vi "Init MFCs Server.vi"(8 "error in":errorcluster) -> (0 "error out":errorcluster, 3 "Alicats":refnum<class "Alicat Device.lvclass">[](array[class]))   [LabVIEW 2015]
uses:
  Devices/Alicat/Session Based/Alicat Device.lvclass
  Controls/MFC Address.ctl
  Reusable/Session APIs/File Access/Config Data/Config Data.lvclass
  Reusable/Session APIs/Serial/Serial Session.lvclass
  Reusable/Session APIs/File Access/Config Data/Config Session.ctl
  Reusable/Session Log/System Log.lvclass
  Reusable/Session Log/System Log.lvclass/System Log.ctl
  Reusable/Session APIs/File Access/Config Data/Config Data.lvclass/Config Data.ctl
  Reusable/Session APIs/Text Communication/Text Device Session.lvclass/Text Device Session.ctl
  Devices/Configurable Device/Configurable Device.lvclass/Configurable Device.ctl
  Devices/Alicat/Session Based/Alicat Device.lvclass/Alicat Device.ctl
  Reusable/Session APIs/Text Communication/Write hSysLog.vi
  Devices/Configurable Device/Write Handle.vi
  Devices/Alicat/Session Based/Accessors/Write Session Handle.vi
  Devices/Alicat/Session Based/Accessors/Write ID.vi
  Reusable/Session Log/Accessors/Write Main Path.vi
  <vilib>/Utility/config.llb/Read Key (String).vi
  <userlib>/_Session Fwk/Session - Root.lvclass
  <vilib>/Utility/config.llb/NI_LVConfig.lvlib
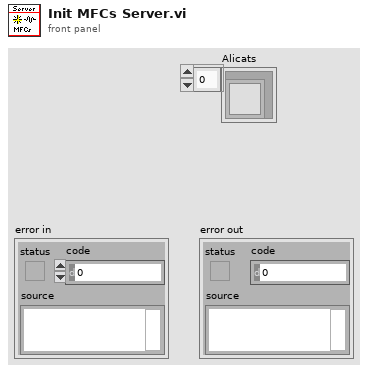
[diagram p1: front panel]
types:
  T1 = typedef "Config Data.lvclass/Config Session.ctl" = refnum<data-value>
  T2 = typedef "MFC Address.ctl" = enum16{"CRDS Purge", "CRDS Thermodenuded", "CRDS Dry", "CRDS Med RH", "CRDS High RH", "PAS Ch 1", "PAS Ch 2", "PAS Ch3", "PAS Ch 4", "PAS Ch 5", "CLAP", "O3", "Pinlet"}
  T3 = typedef "Session - Root.lvclass/Session Handle.ctl" = refnum<data-value>
  T4 = typedef "NI_LVConfig.lvlib/Config Data RefNum.ctl" = refnum<k1>
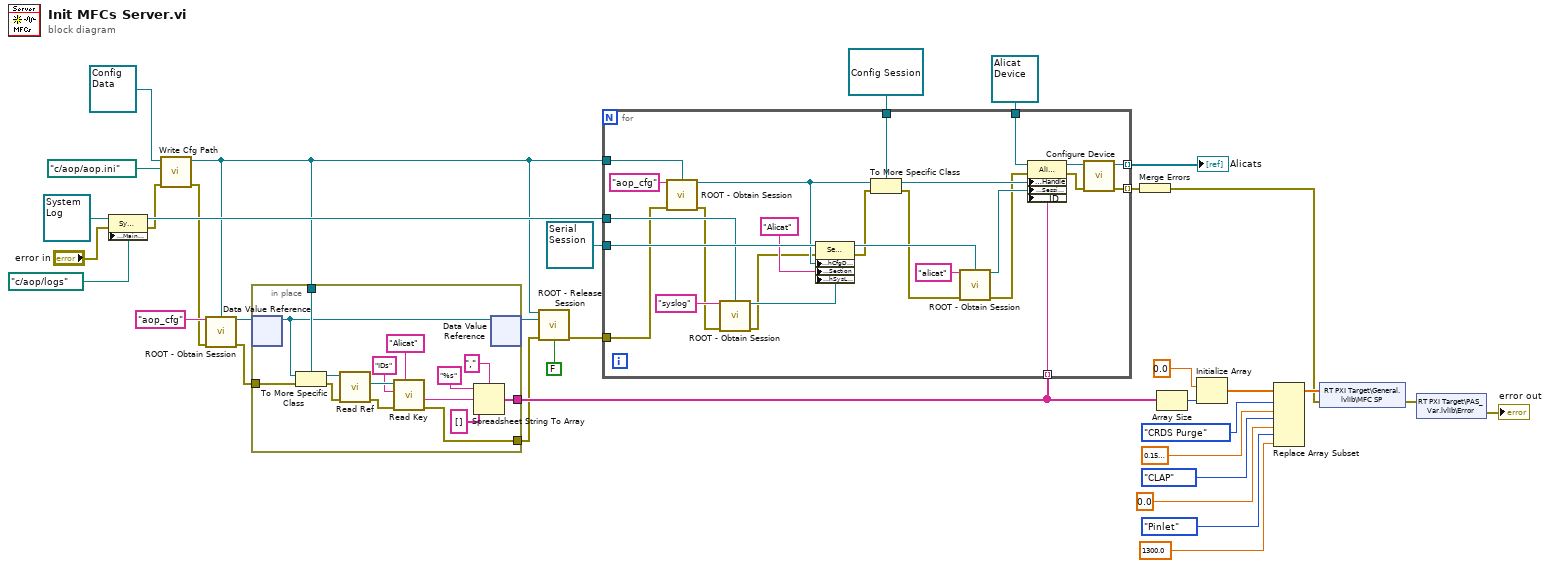
[diagram p0: block diagram]
diagram:
  n1 = property class="Sys Log"(reference=refnum<class "System Log.lvclass"> refnum ("Sys Log"), error in="error in", "Accessors:Main Path"=path "c:/aop/logs" ("Main Path")) -> (reference out=w16:refnum<class "System Log.lvclass">, error out=w2:errorcluster)
  n2 = call "Write Cfg Path.vi"("error in (no error)"=w2, "Cfg Path"=path "c:/aop/aop.ini", "Config Data in"=refnum<class "Config Data.lvclass"> refnum ("Config Data")) -> ("error out"=w1:errorcluster, "Config Data out"=w7:refnum<class "Config Data.lvclass">)  [unwired: 7 in]
  n3 = call <userlib>:"ROOT - Obtain Session.vi"("Session Name ()"="aop_cfg", "OBJ - Session"=w7, "error in (no error)"=w1) -> ("Session Handle"=w10:T3, "error out"=w5:errorcluster)  [unwired: 10 in, 1 out]
  n4 = in-place {
    in-place-border: w7 -> [w50]
    in-place-border: [w41] -> w9
    in-place-border: w5 -> [w37]
    in-place-border: [w36] -> w4
    n5 = in-place-dvr #1(w10) -> (w40:refnum<class "Session - Root.lvclass">)  [unwired: 1 out]
    n6 = To More Specific Class(target class=w50, reference=w40, error in=w37) -> (specific class reference=w49:refnum<class "Config Data.lvclass">, error out=w38:errorcluster)
    n7 = call "Read Ref.vi"("error in (no error)"=w38, "Config Data in"=w49) -> ("error out"=w39:errorcluster, "config data"=w48:T4)  [unwired: 7 in, 1 out]
    n8 = call-poly <vilib>:"Read Key.vi"("section"="Alicat", "error in (no error)"=w39, "key"="IDs", "refnum"=w48) -> ("error out"=w36:errorcluster, "value"=w45:string)  [unwired: 4 in, 2 out]
    n9 = Spreadsheet String To Array(delimiter (Tab)=",", format string="%s", spreadsheet string=w45, array type (2D Dbl)=string[] []) -> (array=w41:string[])
    n10 = in-place-dvr #1(w40) -> (w8:T3)  [unwired: 1 out]
  }
  n11 = call <userlib>:"ROOT - Release Session.vi"("OBJ - Session in"=w7, "Session Handle in"=w8, "error in (no error)"=w4, "force destroy? (F)"=FALSE) -> ("error out"=w3:errorcluster)  [unwired: 10 in, 1 out]
  n12 = for {
    tunnel: w7 -> [w75]
    tunnel: refnum<class "Serial Session.lvclass"> refnum ("Serial Session") -> [w73]
    tunnel: refnum<class "Alicat Device.lvclass"> refnum ("Alicat Device") -> [w69]
    tunnel: T1 refnum ("Handle") -> [w67]
    tunnel: w9 -> [w64] mode=indexing
    tunnel: w16 -> [w63]
    tunnel: [w58] -> w12 mode=indexing
    tunnel: w3 -> [w57]
    tunnel: [w53] -> w15 mode=indexing
    n13 = call <userlib>:"ROOT - Obtain Session.vi"("Session Name ()"="aop_cfg", "OBJ - Session"=w75, "error in (no error)"=w57) -> ("Session Handle"=w68:T3, "error out"=w56:errorcluster)  [unwired: 10 in, 1 out]
    n14 = call <userlib>:"ROOT - Obtain Session.vi"("Session Name ()"="syslog", "OBJ - Session"=w63, "error in (no error)"=w56) -> ("Session Handle"=w61:T3, "error out"=w55:errorcluster)  [unwired: 10 in, 1 out]
    n15 = property class="Serial Session"(reference=w73, error in=w55, "Accessors:hCfgData"=w68, "Accessors:Section"="Alicat" ("Section"), "Accessors:hSysLog"=w61) -> (reference out=w71:refnum<class "Serial Session.lvclass">, error out=w52:errorcluster)
    n16 = To More Specific Class(target class=w67, reference=w68, error in=w52) -> (specific class reference=w65:T1, error out=w51:errorcluster)
    n17 = call <userlib>:"ROOT - Obtain Session.vi"("Session Name ()"="alicat", "OBJ - Session"=w71, "error in (no error)"=w51) -> ("Session Handle"=w66:T3, "error out"=w54:errorcluster)  [unwired: 10 in, 1 out]
    n18 = property class="Alicat Device"(reference=w69, error in=w54, "Accessors:Handle"=w65, "Accessors:Session Handle"=w66, "Accessors:ID"=w64) -> (reference out=w60:refnum<class "Alicat Device.lvclass">, error out=w59:errorcluster)
    n19 = call-dynamic "Configure Device.vi"("error in"=w59, "Alicat Device in"=w60) -> ("error out"=w53:errorcluster, "Alicat Device out"=w58:refnum<class "Alicat Device.lvclass">)  [unwired: 8 in]
  }
  "Alicats" <- w12
  n20 = Merge Errors(w15) -> (w14:errorcluster)
  n21 = Array Size(array=w9) -> (size(s)=w35:i32)
  n22 = Initialize Array(sgl 0.0 ("element"), w35) -> (w33:sgl[])
  n23 = Replace Array Subset(array=w33, new element #1=sgl 0.16 ("CRDS Purge"), index #1=MFC_Address."CRDS Purge" ("Controllers"), new element #2=sgl 0.0 ("new element/subarray"), index #2=MFC_Address."CLAP" ("Controllers"), new element #3=sgl 1300.0 ("new element/subarray"), index #3=MFC_Address."Pinlet" ("Controllers")) -> (w31:sgl[])
  n24 = shared-variable "RT PXI Target\\General.lvlib\\MFC SP"(w31, error in=w14) -> (error out=w29:errorcluster)
  n25 = shared-variable "RT PXI Target\\PAS_Var.lvlib\\Error"(w29) -> (error out=→"error out":errorcluster)  [unwired: 1 in]
